vi "caracterização do ntc.vi"(8 "Resistência":u16(ring) items=["2252", "3000", "5000", "10000", "30000", "100000"], 11 "Temperatura":dbl) -> (2 "R_NTC":dbl)   [LabVIEW 2021]
uses:
  <vilib>/express/express arith-compare/Formula/XNode/ExpressFormulaBlockNode.xnode
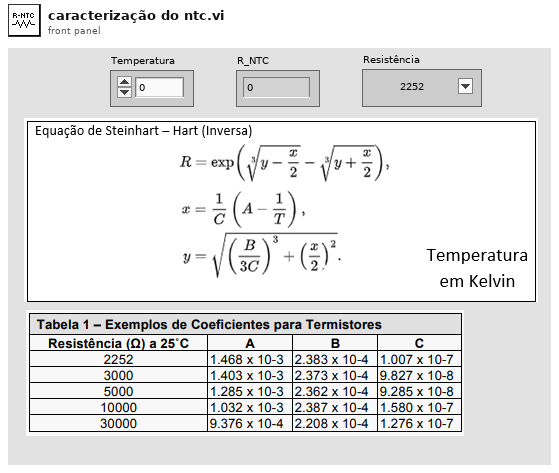
[diagram p1: front panel]
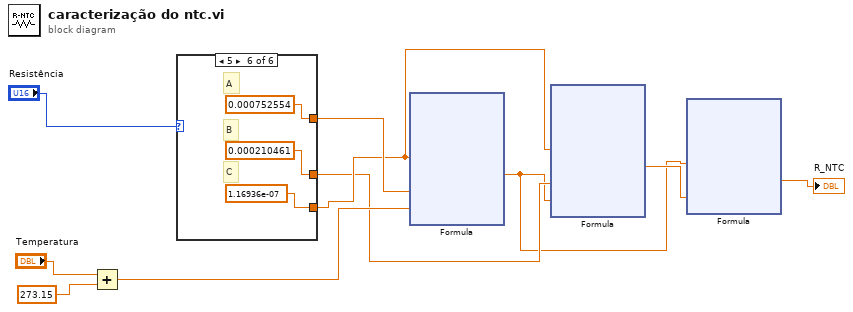
[diagram p0: block diagram]
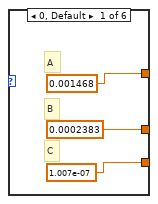
[diagram p2: hidden frame]
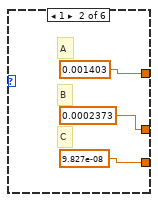
[diagram p3: hidden frame]
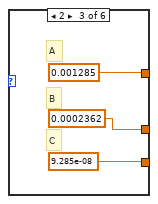
[diagram p4: hidden frame]
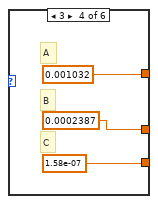
[diagram p5: hidden frame]
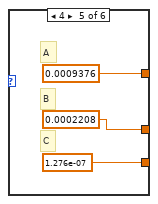
[diagram p6: hidden frame]
diagram:
  n1 = Add(x="Temperatura", y=273.15) -> (x+y=w7:dbl)
  n2 = case shown="5" "Resistência" {
    tunnel: [0.001468 0.001403 0.001285 0.001032 0.0009376 0.000752554] -> w6
    tunnel: [1.007e-07 9.827e-08 9.285e-08 1.58e-07 1.276e-07 1.16936e-07] -> w5
    tunnel: [0.0002383 0.0002373 0.0002362 0.0002387 0.0002208 0.000210461] -> w4
    frame 0, Default {
      # "C"
      # "B"
      # "A"
    }
    frame 1 {
      # "C"
      # "B"
      # "A"
    }
    frame 2 {
      # "C"
      # "B"
      # "A"
    }
    frame 3 {
      # "C"
      # "B"
      # "A"
    }
    frame 4 {
      # "C"
      # "B"
      # "A"
    }
    frame 5 {
      # "C"
      # "B"
      # "A"
    }
  }
  n3 = xnode "Formula"("C"=w5, "A"=w6, "T"=w7) -> ("Result"=w2:dbl)  [unwired: 1 in, 1 out]
  n4 = xnode "Formula"("C"=w5, "B"=w4, "x"=w2) -> ("Result"=w3:dbl)  [unwired: 1 in, 1 out]
  n5 = xnode "Formula"("x"=w2, "y"=w3) -> ("Result"=→"R_NTC":dbl)  [unwired: 1 in, 1 out]
